vi "detections_curve.vi"(11 "timetags":u32[][](array[numeric])) -> (1 "detections":u32[](array[numeric]))   [LabVIEW 2018]
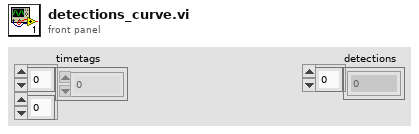
[diagram p1: front panel]
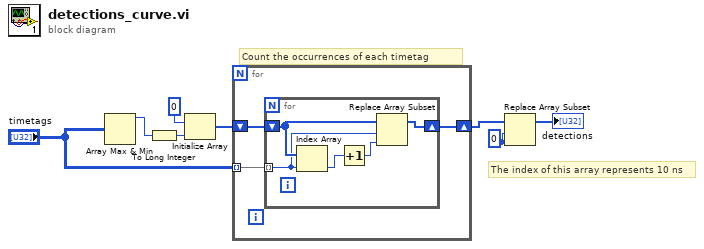
[diagram p0: block diagram]
diagram:
  w1 = 0 ("index")
  # "The index of this array represents 10 ns"
  # "Count the occurrences of each timetag"
  n1 = Array Max & Min(array="timetags") -> (max value=w6:u32)  [unwired: 3 out]
  n2 = To Long Integer(number=w6) -> (32bit integer=w7:i32)
  n3 = Initialize Array(u32 0 ("element"), w7) -> (w4:u32[])
  n4 = for {
    tunnel: "timetags" -> [w11] mode=indexing
    shift-right: [w9] -> w3
    shift-left: w4 -> [w10]
    n5 = for {
      tunnel: w11 -> [w13] mode=indexing
      shift-right: [w12] -> w9
      shift-left: w10 -> [w15]
      n6 = Index Array(array=w15, index=w13) -> (element=w16:u32)
      n7 = Increment(x=w16) -> (x+1=w14:u32)
      n8 = Replace Array Subset(array=w15, new element=w14, index=w13) -> (w12:u32[])
    }
  }
  n9 = Replace Array Subset(array=w3, new element=w1, index=w1) -> (→"detections":u32[])
